vi "Rotate Piece.vi"(8 "Error In":errorcluster caption="Entrée d'erreur", 10 "Move":T5, 11 "Piece Description":T2) -> (0 "Error Out":errorcluster caption="Sortie d'erreur", 1 "New Rotation State":T1, 2 "Rotated Coordinates":T4[](array[typedef]), 3 "Piece Description Out":T2)   [LabVIEW 2017]
uses:
  Controls/Piece Description.ctl
  Controls/Pieces Geometry Names.ctl
  Controls/Coordinates.ctl
  Controls/Rotation State.ctl
  Controls/Moves.ctl
  <vilib>/Analysis/Matrix/Datatypes/RealMatrix.ctl
  <vilib>/Analysis/Matrix/NI_Matrix.lvlib
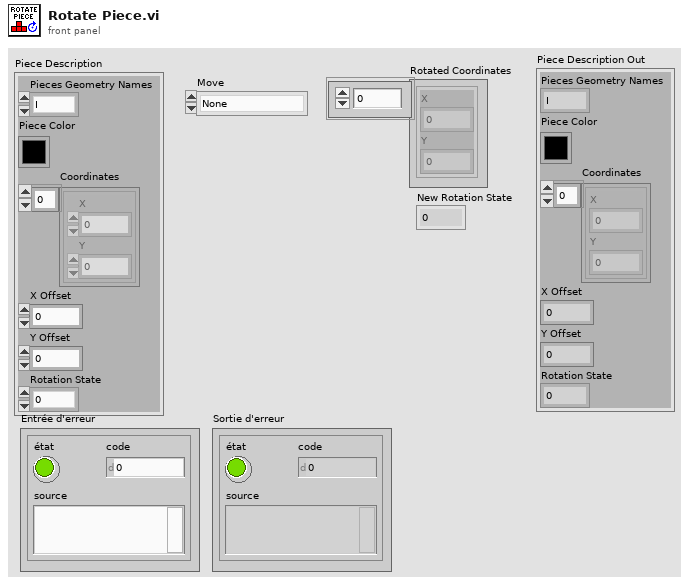
[diagram p1: front panel]
types:
  T1 = typedef "Rotation State.ctl" = enum16{"0", "90", "180", "270"}
  T2 = typedef "Piece Description.ctl" = cluster{"Pieces Geometry Names":T3, "Piece Color":u32, "Coordinates":T4[], "X Offset":i32, "Y Offset":i32, "Rotation State":T1}
  T3 = typedef "Pieces Geometry Names.ctl" = enum16{"I", "O", "T", "L", "J", "Z", "S"}
  T4 = typedef "Coordinates.ctl" = cluster{"X":i32, "Y":i32}
  T5 = typedef "Moves.ctl" = enum16{"None", "Right", "Left", "Step Down", "Go Down", "90 Clockwise", "90 Anti-Clockwise"}
  T6 = typedef "NI_Matrix.lvlib/RealMatrix.ctl" = dbl[][]
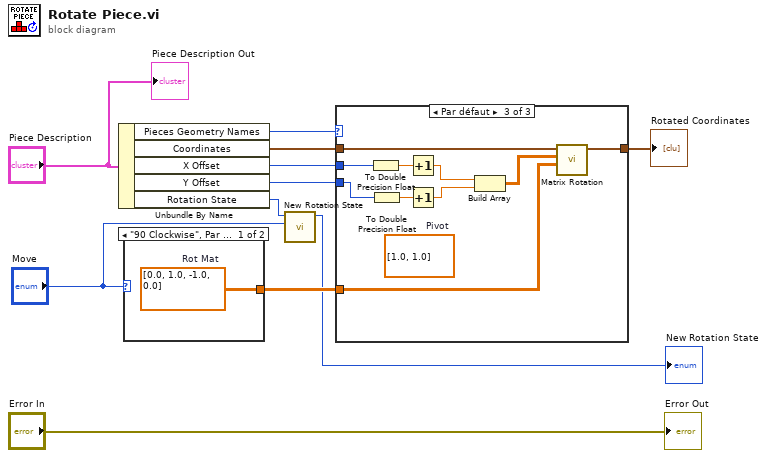
[diagram p0: block diagram]
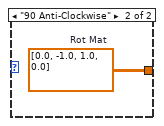
[diagram p2: hidden frame]
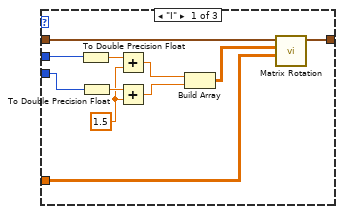
[diagram p3: hidden frame]
diagram:
  n1 = Unbundle By Name("Piece Description") -> ("Pieces Geometry Names"=w11:T3, "Coordinates"=w4:T4[], "X Offset"=w6:i32, "Y Offset"=w5:i32, "Rotation State"=w2:T1)
  n2 = case shown="\"90 Clockwise\", Par défaut" "Move" {
    tunnel: [w12 w13] -> w10
    frame "90 Clockwise", Default {
      w12 = T6 [[0.0, 1.0], [-1.0, 0.0]]  # Rot Mat
    }
    frame "90 Anti-Clockwise" {
      w13 = T6 [[0.0, -1.0], [1.0, 0.0]]  # Rot Mat
    }
  }
  n3 = call "New Rotation State.vi"("Move"="Move", "Rotation State"=w2) -> ("New Rotation State"=→"New Rotation State":T1)  [unwired: 9 in]
  n4 = case shown="Par défaut" w11 {
    tunnel: w4 -> [w22 w25 w35]
    tunnel: [w24 w25 w34] -> w8
    tunnel: w10 -> [w23 _ w33]
    tunnel: w6 -> [w20 _ w28]
    tunnel: w5 -> [w21 _ w27]
    frame "I" {
      w17 = 1.5
      n5 = To Double Precision Float(number=w20) -> (double precision float=w19:dbl)
      n6 = To Double Precision Float(number=w21) -> (double precision float=w18:dbl)
      n7 = Add(x=w19, y=w17) -> (x+y=w16:dbl)
      n8 = Add(x=w18, y=w17) -> (x+y=w15:dbl)
      n9 = Build Array(w16, w15) -> (w14:T6)
      n10 = call "Matrix Rotation.vi"("Rot Mat"=w23, "Pivot"=w14, "Coordinates"=w22) -> ("Rotated Coordinates"=w24:T4[])  [unwired: 7 in, 1 out]
    }
    frame "O" {
    }
    frame Default {
      (unwired) T6 [[1.0], [1.0]]  # Pivot
      n11 = To Double Precision Float(number=w28) -> (double precision float=w32:dbl)
      n12 = To Double Precision Float(number=w27) -> (double precision float=w31:dbl)
      n13 = Increment(x=w32) -> (x+1=w30:dbl)
      n14 = Increment(x=w31) -> (x+1=w29:dbl)
      n15 = Build Array(w30, w29) -> (w26:T6)
      n16 = call "Matrix Rotation.vi"("Rot Mat"=w33, "Pivot"=w26, "Coordinates"=w35) -> ("Rotated Coordinates"=w34:T4[])  [unwired: 7 in, 1 out]
    }
  }
  "Rotated Coordinates" <- w8
  "Error Out" <- "Error In"
  "Piece Description Out" <- "Piece Description"
